vi "close.vi"(8 "error in (no error)":errorcluster, 11 "MOXAIP in":refnum<class "MOXAIP.lvclass">) -> (0 "error out":errorcluster, 3 "MOXAIP out":refnum<class "MOXAIP.lvclass">)   [LabVIEW 2017, in "Serializer.lvlib" / "MOXAIP.lvclass"]
uses:
  MOXAIP.lvclass
  MOXAIP.lvclass/MOXAIP.ctl
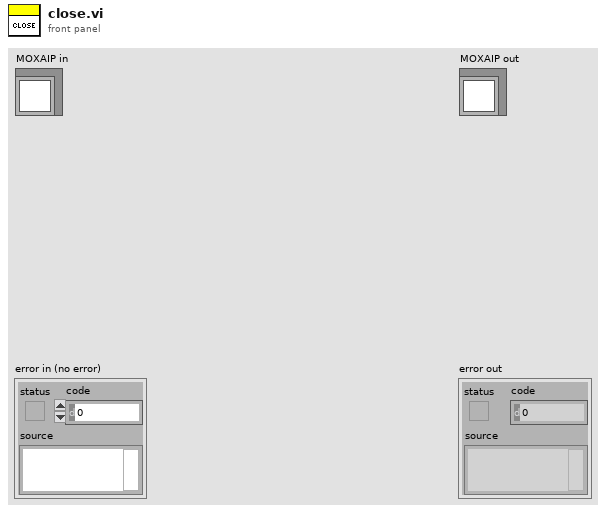
[diagram p1: front panel]
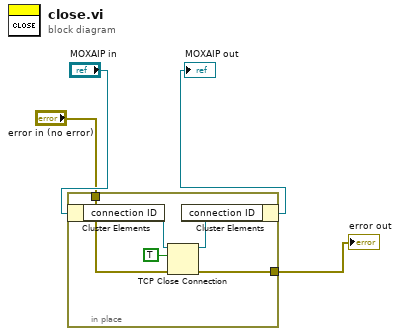
[diagram p0: block diagram]
diagram:
  n1 = in-place {
    in-place-border: "error in (no error)" -> [w6]
    in-place-border: [w5] -> w1
    n2 = in-place-cluster #1("MOXAIP in") -> ("connection ID"=w9:refnum<k5>)
    n3 = TCP Close Connection(connection ID=w9, abort (F)=TRUE, error in (no error)=w6) -> (connection ID out=w7:refnum<k5>, error out=w5:errorcluster)
    n4 = in-place-cluster #1("connection ID"=w7) -> (→"MOXAIP out":refnum<class "MOXAIP.lvclass">)
  }
  "error out" <- w1
